vi "users logout user.vi"(6 "Current User":T2, 7 "HTTP Header (\"\")":string, 8 "error in (no error)":errorcluster, 10 "Username to Logout (\"\")":string, 11 "Connection Refnum":T1) -> (0 "error out":errorcluster, 3 "Connection Refnum":T1, 5 "new HTTP Header":string)   [LabVIEW 2011]
uses:
  server/database/Users/User Record.ctl
  SI.LIB/ODBC/SQL Controls/Connection Refnum.ctl
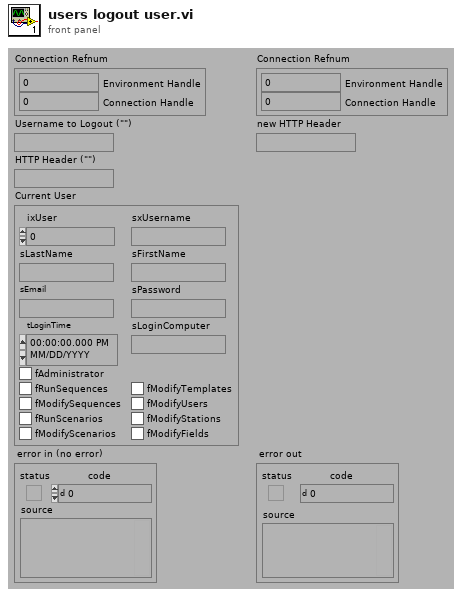
[diagram p1: front panel]
types:
  T1 = typedef "Connection Refnum.ctl" = cluster{"Environment Handle":i32, "Connection Handle":i32}
  T2 = typedef "User Record.ctl" = cluster{"ixUser":i32, "sxUsername":string, "sLastName":string, "sFirstName":string, "sEmail":string, "sPassword":string, "tLoginTime":timestamp, "sLoginComputer":string, "fAdministrator":bool, "fRunSequences":bool, "fModifySequences":bool, "fRunScenarios":bool, "fModifyScenarios":bool, "fModifyTemplates":bool, "fModifyUsers":bool, "fModifyStations":bool, "fModifyFields":bool}
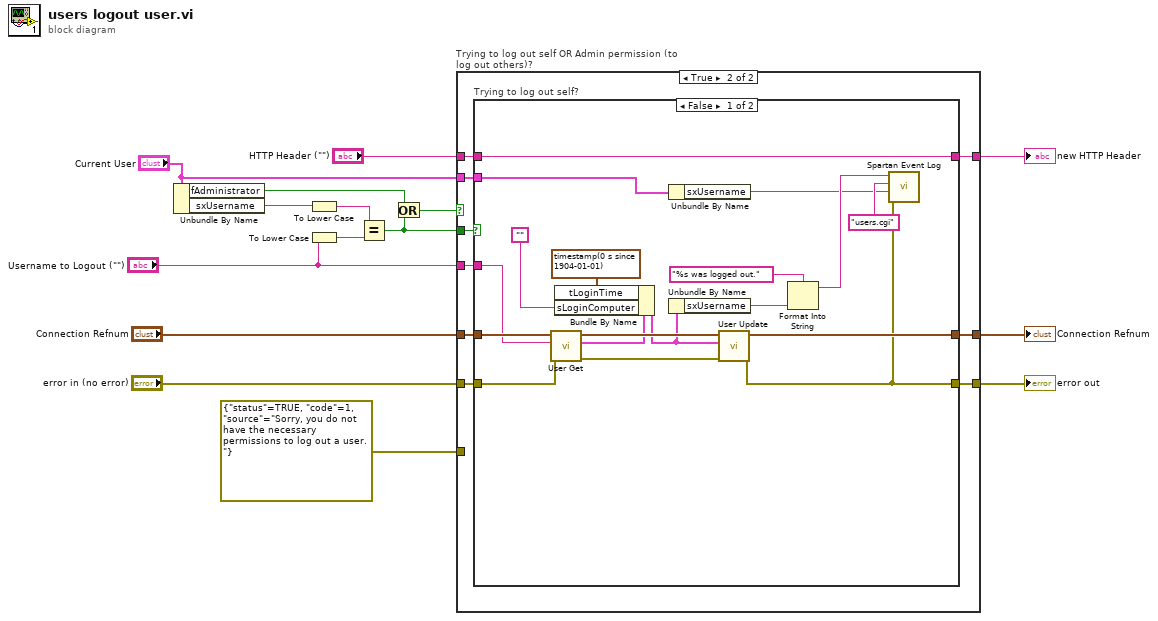
[diagram p0: block diagram]
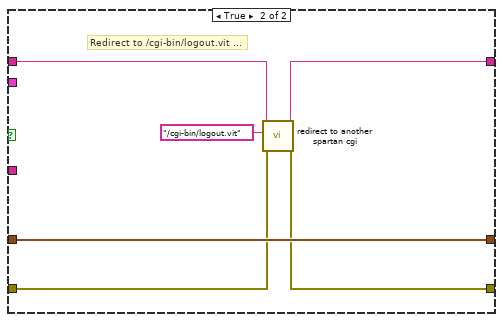
[diagram p3: hidden frame]
diagram:
  n1 = Unbundle By Name("Current User") -> ("fAdministrator"=w7:bool, "sxUsername"=w9:string)
  n2 = To Lower Case(string=w9) -> (all lower case string=w8:string)
  n3 = To Lower Case(string="Username to Logout (\"\")") -> (all lower case string=w10:string)
  n4 = Equal?(x=w8, y=w10) -> (x = y?=w3:bool)
  n5 = Or(x=w7, y=w3) -> (x .or. y?=w6:bool)
  n6 = case "Trying to log out self OR Admin permission (to log out others)?" shown="True" w6 {
    tunnel: "error in (no error)" -> [_ w27]
    tunnel: "Connection Refnum" -> [w18 w26]
    tunnel: [w18 w25] -> w13
    tunnel: [w17 w24] -> w12
    tunnel: "Username to Logout (\"\")" -> [_ w23]
    tunnel: errorcluster {"status"=TRUE, "code"=1, "source"="Sorry, you do not have the necessary permissions to log out a user."} ("error out") -> [w17 _]
    tunnel: "Current User" -> [_ w21]
    tunnel: w3 -> [_ w22]
    tunnel: [w16 w20] -> w1
    tunnel: "HTTP Header (\"\")" -> [w16 w19]
    frame False {
    }
    frame True {
      n7 = case "Trying to log out self?" shown="False" w22 {
        tunnel: w27 -> [w42 w50]
        tunnel: w26 -> [w41 w51]
        tunnel: [w40 w51] -> w25
        tunnel: [w37 w49] -> w24
        tunnel: w23 -> [w38 _]
        tunnel: w21 -> [w31 _]
        tunnel: [w29 w48] -> w20
        tunnel: w19 -> [w29 w47]
        frame False {
          n8 = call "User Get.vi"("error in (no error)"=w42, "sxUsername (\"\")"=w38, "Connection Refnum"=w41) -> ("error out"=w44:errorcluster, "User"=w43:T2, "Connection Refnum"=w45:T1)  [unwired: 6 out]
          n9 = Bundle By Name(cluster=w43, "tLoginTime"=timestamp(0 s since 1904-01-01), "sLoginComputer"="") -> (w36:T2)
          n10 = Unbundle By Name(w31) -> ("sxUsername"=w30:string)
          n11 = Unbundle By Name(w36) -> ("sxUsername"=w34:string)
          n12 = call "User Update.vi"("error in (no error)"=w44, "User Record"=w36, "Connection Refnum"=w45) -> ("error out"=w37:errorcluster, "dup Connection Refnum"=w40:T1)  [unwired: 7 out]
          n13 = Format Into String(format string="%s was logged out.", w34) -> (resulting string=w33:string)  [unwired: 2 in, 1 out]
          n14 = call "Spartan Event Log.vi"("error in (no error)"=w37, "username (\"\")"=w30, "module (\"\")"="users.cgi", "message (\"\")"=w33) -> ()  [unwired: 1 in, 4 out]
        }
        frame True {
          # "Redirect to /cgi-bin/logout.vit ..."
          n15 = call "redirect to another spartan cgi.vi"("error in (no error)"=w50, "New URL (/cgi-bin/testing.vit)"="/cgi-bin/logout.vit", "Original Header In (to be replaced)"=w47) -> ("error out"=w49:errorcluster, "Redirection Header"=w48:string)  [unwired: 1 in, 6 out]
        }
      }
    }
  }
  "error out" <- w12
  "Connection Refnum" <- w13
  "new HTTP Header" <- w1
